vi "DisplayJson.vi"(11 "JSON String In":string="[{\"version\":\"1.0.0\",\"header\":{\"creationDate\":\"2022-06-03T00:00:00\",\"remarks\":\"\",\"serialNumber\":\"98172\",\"productNumber\":\"123021.1804\",\"productType\":\"PAA-9L\",\"pressureType\":2,\"productSeries\":\"9L\",\"compensatedTemperatureRange\":{\"min\":-10.0,\"max\":80.0,\"unit\":4},\"compensatedPressureRange\":{\"min\":0.0,\"max\":0.35,\"unit\":3},\"electricSupply\":{\"magnitude\":1.0,\"unit\":18},\"orderNumber\":9990266,\"orderPosition\":3,\"orderTargetDispatchDate\":\"2022-06-02T00:00:00+00:00\",\"customerName\":\"DemoData Inc.\",\"customerNumber\":12345678,\"customerOrderNumber\":\"Cust-9990266-123\",\"customerReferenceNumber\":\"\",\"customerProductT...") -> ()   [LabVIEW 2017] (continued)
magnitude\":59.8651,\"unit\":4},\"supply\":{\"magnitude\":1.0,\"unit\":18}},\"raw\":{\"signal\":{\"magnitude\":64.467783206,\"unit\":22},\"bridgeResistance\":{\"magnitude\":3852.3455546,\"unit\":28}},\"compensated\":{\"mathematicalModels\":{\"MM0123\":{\"pressure\":{\"output\":{\"magnitude\":0.349985,\"unit\":3},\"error\":{\"magnitude\":-0.0019717653,\"unit\":7}},\"temperature\":{\"output\":{\"magnitude\":59.9371,\"unit\":4},\"error\":{\"magnitude\":0.071974206,\"unit\":4}}}}}},{\"reference\":\"F_12300_XX_0000098765\",\"environmentTarget\":{\"pressure\":{\"magnitude\":0.03,\"unit\":3},\"temperature\":{\"magnitude\":80.0,\"unit\":4}},\"environment\":{\"pressure\":{\"magnitude\":0.0299952,\"unit\":3},\"temperature\":{\"magnitude\":79.9513,\"unit\":4},\"supply\":{\"magnitude\":1.0,\"unit\":18}},\"raw\":{\"signal\":{\"magnitude\":20.009624769,\"unit\":22},\"bridgeResistance\":{\"magnitude\":4076.9393183,\"unit\":28}},\"compensated\":{\"mathematicalModels\":{\"MM0123\":{\"pressure\":{\"output\":{\"magnitude\":0.0300118,\"unit\":3},\"error\":{\"magnitude\":0.0047428932,\"unit\":7}},\"temperature\":{\"output\":{\"magnitude\":80.0429,\"unit\":4},\"error\":{\"magnitude\":0.091598008,\"unit\":4}}}}}},{\"reference\":\"F_12300_XX_0000098765\",\"environmentTarget\":{\"pressure\":{\"magnitude\":0.11,\"unit\":3},\"temperature\":{\"magnitude\":80.0,\"unit\":4}},\"environment\":{\"pressure\":{\"magnitude\":0.110003,\"unit\":3},\"temperature\":{\"magnitude\":79.9513,\"unit\":4},\"supply\":{\"magnitude\":1.0,\"unit\":18}},\"raw\":{\"signal\":{\"magnitude\":31.586032437,\"unit\":22},\"bridgeResistance\":{\"magnitude\":4072.4664155,\"unit\":28}},\"compensated\":{\"mathematicalModels\":{\"MM0123\":{\"pressure\":{\"output\":{\"magnitude\":0.109961,\"unit\":3},\"error\":{\"magnitude\":-0.011912582,\"unit\":7}},\"temperature\":{\"output\":{\"magnitude\":80.0462,\"unit\":4},\"error\":{\"magnitude\":0.094860315,\"unit\":4}}}}}},{\"reference\":\"F_12300_XX_0000098765\",\"environmentTarget\":{\"pressure\":{\"magnitude\":0.19,\"unit\":3},\"temperature\":{\"magnitude\":80.0,\"unit\":4}},\"environment\":{\"pressure\":{\"magnitude\":0.189995,\"unit\":3},\"temperature\":{\"magnitude\":79.9513,\"unit\":4},\"supply\":{\"magnitude\":1.0,\"unit\":18}},\"raw\":{\"signal\":{\"magnitude\":43.149115129,\"unit\":22},\"bridgeResistance\":{\"magnitude\":4068.082853,\"unit\":28}},\"compensated\":{\"mathematicalModels\":{\"MM0123\":{\"pressure\":{\"output\":{\"magnitude\":0.190002,\"unit\":3},\"error\":{\"magnitude\":0.0020917834,\"unit\":7}},\"temperature\":{\"output\":{\"magnitude\":80.0546,\"unit\":4},\"error\":{\"magnitude\":0.10324897,\"unit\":4}}}}}},{\"reference\":\"F_12300_XX_0000098765\",\"environmentTarget\":{\"pressure\":{\"magnitude\":0.27,\"unit\":3},\"temperature\":{\"magnitude\":80.0,\"unit\":4}},\"environment\":{\"pressure\":{\"magnitude\":0.270005,\"unit\":3},\"temperature\":{\"magnitude\":79.9513,\"unit\":4},\"supply\":{\"magnitude\":1.0,\"unit\":18}},\"raw\":{\"signal\":{\"magnitude\":54.683724116,\"unit\":22},\"bridgeResistance\":{\"magnitude\":4063.7153683,\"unit\":28}},\"compensated\":{\"mathematicalModels\":{\"MM0123\":{\"pressure\":{\"output\":{\"magnitude\":0.270035,\"unit\":3},\"error\":{\"magnitude\":0.0086059364,\"unit\":7}},\"temperature\":{\"output\":{\"magnitude\":80.0606,\"unit\":4},\"error\":{\"magnitude\":0.10926909,\"unit\":4}}}}}},{\"reference\":\"F_12300_XX_0000098765\",\"environmentTarget\":{\"pressure\":{\"magnitude\":0.35,\"unit\":3},\"temperature\":{\"magnitude\":80.0,\"unit\":4}},\"environment\":{\"pressure\":{\"magnitude\":0.350001,\"unit\":3},\"temperature\":{\"magnitude\":79.9513,\"unit\":4},\"supply\":{\"magnitude\":1.0,\"unit\":18}},\"raw\":{\"signal\":{\"magnitude\":66.178985809,\"unit\":22},\"bridgeResistance\":{\"magnitude\":4059.3928573,\"unit\":28}},\"compensated\":{\"mathematicalModels\":{\"MM0123\":{\"pressure\":{\"output\":{\"magnitude\":0.349984,\"unit\":3},\"error\":{\"magnitude\":-0.0048720874,\"unit\":7}},\"temperature\":{\"output\":{\"magnitude\":80.0663,\"unit\":4},\"error\":{\"magnitude\":0.114986,\"unit\":4}}}}}}]},{\"version\":\"1.0.0\",\"header\":{\"creationDate\":\"2022-06-03T00:00:00\",\"remarks\":\"\",\"serialNumber\":\"98030\",\"productNumber\":\"123021.1804\",\"productType\":\"PAA-9L\",\"pressureType\":2,\"productSeries\":\"9L\",\"compensatedTemperatureRange\":{\"min\":-10.0,\"max\":80.0,\"unit\":4},\"compensatedPressureRange\":{\"min\":0.0,\"max\":0.35,\"unit\":3},\"electricSupply\":{\"magnitude\":1.0,\"unit\":18},\"orderNumber\":9990266,\"orderPosition\":3,\"orderTargetDispatchDate\":\"2022-06-02T00:00:00+00:00\",\"customerName\":\"DemoData Inc.\",\"customerNumber\":12345678,\"customerOrderNumber\":\"Cust-9990266-123\",\"customerReferenceNumber\":\"\",\"customerProductType\":\"123021-1804 Rev.AA\"},\"compensationMethods\":{\"mathematicalModels\":{\"MM0123\":{\"modelType\":\"MM0123\",\"productNumber\":\"000000.0000\",\"compensatedTemperatureRange\":{\"min\":-10.0,\"max\":80.0,\"unit\":4},\"compensatedPressureRange\":{\"min\":0.0,\"max\":0.35,\"unit\":3},\"electricSupply\":{\"magnitude\":1.0,\"unit\":18},\"parts\":{\"pressure\":{\"inputs\":[\"Sig\",\"R\"],\"output\":\"P\",\"description\":\"P = f(Sig,R)\",\"coefficients\":[[3.91051610792,-0.00396303697808,1.49281608913E-06,-2.51964333732E-10,1.59626202738E-14],[-0.118371633509,0.000126551102362,-4.7723277619E-08,7.99004276927E-12,-5.02310435685E-16],[-0.000301862256289,3.5208950299E-07,-1.51215801138E-10,2.85596859923E-14,-2.00879963271E-18]]},\"temperature\":{\"inputs\":[\"R\",\"Sig\"],\"output\":\"T\",\"description\":\"T = f(R,Sig)\",\"coefficients\":[[-7800.26845732,-7.96154289458,0.0704333830142],[7.62753908696,0.00996321268213,-8.05974057259E-05],[-0.00286192784163,-4.51133002231E-06,3.42637785226E-08],[4.86703234067E-07,8.89561295675E-10,-6.42476105441E-12],[-3.12400283304E-11,-6.46081048648E-14,4.48929986852E-16]]}}}}},\"measurements\":[{\"reference\":\"F_12300_XX_0000098765\",\"environmentTarget\":{\"pressure\":{\"magnitude\":0.03,\"unit\":3},\"temperature\":{\"magnitude\":-10.0,\"unit\":4}},\"environment\":{\"pressure\":{\"magnitude\":0.0300053,\"unit\":3},\"temperature\":{\"magnitude\":-10.7286,\"unit\":4},\"supply\":{\"magnitude\":1.0,\"unit\":18}},\"raw\":{\"signal\":{\"magnitude\":14.318461418,\"unit\":22},\"bridgeResistance\":{\"magnitude\":3289.5907634,\"unit\":28}},\"compensated\":{\"mathematicalModels\":{\"MM0123\":{\"pressure\":{\"output\":{\"magnitude\":0.0300169,\"unit\":3},\"error\":{\"magnitude\":0.0033129561,\"unit\":7}},\"temperature\":{\"output\":{\"magnitude\":-10.8169,\"unit\":4},\"error\":{\"magnitude\":-0.089267989,\"unit\":4}}}}}},{\"reference\":\"F_12300_XX_0000098765\",\"environmentTarget\":{\"pressure\":{\"magnitude\":0.11,\"unit\":3},\"temperature\":{\"magnitude\":-10.0,\"unit\":4}},\"environment\":{\"pressure\":{\"magnitude\":0.10999,\"unit\":3},\"temperature\":{\"magnitude\":-10.7286,\"unit\":4},\"supply\":{\"magnitude\":1.0,\"unit\":18}},\"raw\":{\"signal\":{\"magnitude\":25.459617511,\"unit\":22},\"bridgeResistance\":{\"magnitude\":3284.2812107,\"unit\":28}},\"compensated\":{\"mathematicalModels\":{\"MM0123\":{\"pressure\":{\"output\":{\"magnitude\":0.109962,\"unit\":3},\"error\":{\"magnitude\":-0.0079150781,\"unit\":7}},\"temperature\":{\"output\":{\"magnitude\":-10.8249,\"unit\":4},\"error\":{\"magnitude\":-0.096259313,\"unit\":4}}}}}},{\"reference\":\"F_12300_XX_0000098765\",\"environmentTarget\":{\"pressure\":{\"magnitude\":0.19,\"unit\":3},\"temperature\":{\"magnitude\":-10.0,\"unit\":4}},\"environment\":{\"pressure\":{\"magnitude\":0.190001,\"unit\":3},\"temperature\":{\"magnitude\":-10.7286,\"unit\":4},\"supply\":{\"magnitude\":1.0,\"unit\":18}},\"raw\":{\"signal\":{\"magnitude\":36.571102004,\"unit\":22},\"bridgeResistance\":{\"magnitude\":3280.172315,\"unit\":28}},\"compensated\":{\"mathematicalModels\":{\"MM0123\":{\"pressure\":{\"output\":{\"magnitude\":0.190009,\"unit\":3},\"error\":{\"magnitude\":0.0024238375,\"unit\":7}},\"temperature\":{\"output\":{\"magnitude\":-10.8183,\"unit\":4},\"error\":{\"magnitude\":-0.089645595,\"unit\":4}}}}}},{\"reference\":\"F_12300_XX_0000098765\",\"environmentTarget\":{\"pressure\":{\"magnitude\":0.27,\"unit\":3},\"temperature\":{\"magnitude\":-10.0,\"unit\":4}},\"environment\":{\"pressure\":{\"magnitude\":0.270006,\"unit\":3},\"temperature\":{\"magnitude\":-10.7286,\"unit\":4},\"supply\":{\"magnitude\":1.0,\"unit\":18}},\"raw\":{\"signal\":{\"magnitude\":47.63478106,\"unit\":22},\"bridgeResistance\":{\"magnitude\":3276.1315246,\"unit\":28}},\"compensated\":{\"mathematicalModels\":{\"MM0123\":{\"pressure\":{\"output\":{\"magnitude\":0.270034,\"unit\":3},\"error\":{\"magnitude\":0.0080862094,\"unit\":7}},\"temperature\":{\"output\":{\"magnitude\":-10.8182,\"unit\":4},\"error\":{\"magnitude\":-0.089598768,\"unit\":4}}}}}},{\"reference\":\"F_12300_XX_0000098765\",\"environmentTarget\":{\"pressure\":{\"magnitude\":0.35,\"unit\":3},\"temperature\":{\"magnitude\":-10.0,\"unit\":4}},\"environment\":{\"pressure\":{\"magnitude\":0.35,\"unit\":3},\"temperature\":{\"magnitude\":-10.7286,\"unit\":4},\"supply\":{\"magnitude\":1.0,\"unit\":18}},\"raw\":{\"signal\":{\"magnitude\":58.644972732,\"unit\":22},\"bridgeResistance\":{\"magnitude\":3272.1742491,\"unit\":28}},\"compensated\":{\"mathematicalModels\":{\"MM0123\":{\"pressure\":{\"output\":{\"magnitude\":0.349995,\"unit\":3},\"error\":{\"magnitude\":-0.0015198512,\"unit\":7}},\"temperature\":{\"output\":{\"magnitude\":-10.823,\"unit\":4},\"error\":{\"magnitude\":-0.094366794,\"unit\":4}}}}}},{\"reference\":\"F_12300_XX_0000098765\",\"environmentTarget\":{\"pressure\":{\"magnitude\":0.03,\"unit\":3},\"temperature\":{\"magnitude\":0.0,\"unit\":4}},\"environment\":{\"pressure\":{\"magnitude\":0.0299991,\"unit\":3},\"temperature\":{\"magnitude\":-0.629962,\"unit\":4},\"supply\":{\"magnitude\":1.0,\"unit\":18}},\"raw\":{\"signal\":{\"magnitude\":14.719120521,\"unit\":22},\"bridgeResistance\":{\"magnitude\":3358.468982,\"unit\":28}},\"compensated\":{\"mathematicalModels\":{\"MM0123\":{\"pressure\":{\"output\":{\"magnitude\":0.0300133,\"unit\":3},\"error\":{\"magnitude\":0.0040708695,\"unit\":7}},\"temperature\":{\"output\":{\"magnitude\":-0.731686,\"unit\":4},\"error\":{\"magnitude\":-0.10172384,\"unit\":4}}}}}},{\"reference\":\"F_12300_XX_0000098765\",\"environmentTarget\":{\"pressure\":{\"magnitude\":0.11,\"unit\":3},\"temperature\":{\"magnitude\":0.0,\"unit\":4}},\"environment\":{\"pressure\":{\"magnitude\":0.110012,\"unit\":3},\"temperature\":{\"magnitude\":-0.629962,\"unit\":4},\"supply\":{\"magnitude\":1.0,\"unit\":18}},\"raw\":{\"signal\":{\"magnitude\":25.832280563,\"unit\":22},\"bridgeResistance\":{\"magnitude\":3354.2253146,\"unit\":28}},\"compensated\":{\"mathematicalModels\":{\"MM0123\":{\"pressure\":{\"output\":{\"magnitude\":0.109979,\"unit\":3},\"error\":{\"magnitude\":-0.0093436435,\"unit\":7}},\"temperature\":{\"output\":{\"magnitude\":-0.731795,\"unit\":4},\"error\":{\"magnitude\":-0.10183319,\"unit\":4}}}}}},{\"reference\":\"F_12300_XX_0000098765\",\"environmentTarget\":{\"pressure\":{\"magnitude\":0.19,\"unit\":3},\"temperature\":{\"magnitude\":0.0,\"unit\":4}},\"environment\":{\"pressure\":{\"magnitude\":0.190005,\"unit\":3},\"temperature\":{\"magnitude\":-0.629962,\"unit\":4},\"supply\":{\"magnitude\":1.0,\"unit\":18}},\"raw\":{\"signal\":{\"magnitude\":36.911420503,\"unit\":22},\"bridgeResistance\":{\"magnitude\":3350.0635874,\"unit\":28}},\"compensated\":{\"mathematicalModels\":{\"MM0123\":{\"pressure\":{\"output\":{\"magnitude\":0.190007,\"unit\":3},\"error\":{\"magnitude\":0.00070119695,\"unit\":7}},\"temperature\":{\"output\":{\"magnitude\":-0.733503,\"unit\":4},\"error\":{\"magnitude\":-0.10354162,\"unit\":4}}}}}},{\"reference\":\"F_12300_XX_0000098765\",\"environmentTarget\":{\"pressure\":{\"magnitude\":0.27,\"unit\":3},\"temperature\":{\"magnitude\":0.0,\"unit\":4}},\"environment\":{\"pressure\":{\"magnitude\":0.270005,\"unit\":3},\"temperature\":{\"magnitude\":-0.629962,\"unit\":4},\"supply\":{\"magnitude\":1.0,\"unit\":18}},\"raw\":{\"signal\":{\"magnitude\":47.944742767,\"unit\":22},\"bridgeResistance\":{\"magnitude\":3345.9709897,\"unit\":28}},\"compensated\":{\"mathematicalModels\":{\"MM0123\":{\"pressure\":{\"output\":{\"magnitude\":0.270014,\"unit\":3},\"error\":{\"magnitude\":0.0025000508,\"unit\":7}},\"temperature\":{\"output\":{\"magnitude\":-0.739521,\"unit\":4},\"error\":{\"magnitude\":-0.10955897,\"unit\":4}}}}}},{\"reference\":\"F_12300_XX_0000098765\",\"environmentTarget\":{\"pressure\":{\"magnitude\":0.35,\"unit\":3},\"temperature\":{\"magnitude\":0.0,\"unit\":4}},\"environment\":{\"pressure\":{\"magnitude\":0.350001,\"unit\":3},\"temperature\":{\"magnitude\":-0.629962,\"unit\":4},\"supply\":{\"magnitude\":1.0,\"unit\":18}},\"raw\":{\"signal\":{\"magnitude\":58.929179764,\"unit\":22},\"bridgeResistance\":{\"magnitude\":3342.0076022,\"unit\":28}},\"compensated\":{\"mathematicalModels\":{\"MM0123\":{\"pressure\":{\"output\":{\"magnitude\":0.349974,\"unit\":3},\"error\":{\"magnitude\":-0.0077921223,\"unit\":7}},\"temperature\":{\"output\":{\"magnitude\":-0.741948,\"unit\":4},\"error\":{\"magnitude\":-0.1129859,\"unit\":4}}}}}},{\"reference\":\"F_12300_XX_0000098765\",\"environmentTarget\":{\"pressure\":{\"magnitude\":0.03,\"unit\":3},\"temperature\":{\"magnitude\":20.0,\"unit\":4}},\"environment\":{\"pressure\":{\"magnitude\":0.0300045,\"unit\":3},\"temperature\":{\"magnitude\":19.5509,\"unit\":4},\"supply\":{\"magnitude\":1.0,\"unit\":18}},\"raw\":{\"signal\":{\"magnitude\":15.541489722,\"unit\":22},\"bridgeResistance\":{\"magnitude\":3515.4448937,\"unit\":28}},\"compensated\":{\"mathematicalModels\":{\"MM0123\":{\"pressure\":{\"output\":{\"magnitude\":0.0300159,\"unit\":3},\"error\":{\"magnitude\":0.003267515,\"unit\":7}},\"temperature\":{\"output\":{\"magnitude\":19.5547,\"unit\":4},\"error\":{\"magnitude\":0.0038291876,\"unit\":4}}}}}},{\"reference\":\"F_12300_XX_0000098765\",\"environmentTarget\":{\"pressure\":{\"magnitude\":0.11,\"unit\":3},\"temperature\":{\"magnitude\":20.0,\"unit\":4}},\"environment\":{\"pressure\":{\"magnitude\":0.109996,\"unit\":3},\"temperature\":{\"magnitude\":19.5509,\"unit\":4},\"supply\":{\"magnitude\":1.0,\"unit\":18}},\"raw\":{\"signal\":{\"magnitude\":26.644230328,\"unit\":22},\"bridgeResistance\":{\"magnitude\":3511.171863,\"unit\":28}},\"compensated\":{\"mathematicalModels\":{\"MM0123\":{\"pressure\":{\"output\":{\"magnitude\":0.109975,\"unit\":3},\"error\":{\"magnitude\":-0.005894568,\"unit\":7}},\"temperature\":{\"output\":{\"magnitude\":19.5469,\"unit\":4},\"error\":{\"magnitude\":-0.0039398524,\"unit\":4}}}}}},{\"reference\":\"F_12300_XX_0000098765\",\"environmentTarget\":{\"pressure\":{\"magnitude\":0.19,\"unit\":3},\"temperature\":{\"magnitude\":20.0,\"unit\":4}},\"environment\":{\"pressure\":{\"magnitude\":0.189992,\"unit\":3},\"temperature\":{\"magnitude\":19.5509,\"unit\":4},\"supply\":{\"magnitude\":1.0,\"unit\":18}},\"raw\":{\"signal\":{\"magnitude\":37.718116681,\"unit\":22},\"bridgeResistance\":{\"magnitude\":3507.0336187,\"unit\":28}},\"compensated\":{\"mathematicalModels\":{\"MM0123\":{\"pressure\":{\"output\":{\"magnitude\":0.190001,\"unit\":3},\"error\":{\"magnitude\":0.0026963766,\"unit\":7}},\"temperature\":{\"output\":{\"magnitude\":19.5474,\"unit\":4},\"error\":{\"magnitude\":-0.0034972219,\"unit\":4}}}}}},{\"reference\":\"F_12300_XX_0000098765\",\"environmentTarget\":{\"pressure\":{\"magnitude\":0.27,\"unit\":3},\"temperature\":{\"magnitude\":20.0,\"unit\":4}},\"environment\":{\"pressure\":{\"magnitude\":0.269996,\"unit\":3},\"temperature\":{\"magnitude\":19.5509,\"unit\":4},\"supply\":{\"magnitude\":1.0,\"unit\":18}},\"raw\":{\"signal\":{\"magnitude\":48.753140854,\"unit\":22},\"bridgeResistance\":{\"magnitude\":3502.9189005,\"unit\":28}},\"compensated\":{\"mathematicalModels\":{\"MM0123\":{\"pressure\":{\"output\":{\"magnitude\":0.270027,\"unit\":3},\"error\":{\"magnitude\":0.0087365389,\"unit\":7}},\"temperature\":{\"output\":{\"magnitude\":19.5419,\"unit\":4},\"error\":{\"magnitude\":-0.0089498086,\"unit\":4}}}}}},{\"reference\":\"F_12300_XX_0000098765\",\"environmentTarget\":{\"pressure\":{\"magnitude\":0.35,\"unit\":3},\"temperature\":{\"magnitude\":20.0,\"unit\":4}},\"environment\":{\"pressure\":{\"magnitude\":0.350008,\"unit\":3},\"temperature\":{\"magnitude\":19.5509,\"unit\":4},\"supply\":{\"magnitude\":1.0,\"unit\":18}},\"raw\":{\"signal\":{\"magnitude\":59.744665253,\"unit\":22},\"bridgeResistance\":{\"magnitude\":3498.9179563,\"unit\":28}},\"compensated\":{\"mathematicalModels\":{\"MM0123\":{\"pressure\":{\"output\":{\"magnitude\":0.350014,\"unit\":3},\"error\":{\"magnitude\":0.0016130378,\"unit\":7}},\"temperature\":{\"output\":{\"magnitude\":19.5411,\"unit\":4},\"error\":{\"magnitude\":-0.0098247912,\"unit\":4}}}}}},{\"reference\":\"F_12300_XX_0000098765\",\"environmentTarget\":{\"pressure\":{\"magnitude\":0.03,\"unit\":3},\"temperature\":{\"magnitude\":40.0,\"unit\":4}},\"environment\":{\"pressure\":{\"magnitude\":0.0300059,\"unit\":3},\"temperature\":{\"magnitude\":39.7284,\"unit\":4},\"supply\":{\"magnitude\":1.0,\"unit\":18}},\"raw\":{\"signal\":{\"magnitude\":16.399203422,\"unit\":22},\"bridgeResistance\":{\"magnitude\":3691.7829758,\"unit\":28}},\"compensated\":{\"mathematicalModels\":{\"MM0123\":{\"pressure\":{\"output\":{\"magnitude\":0.03002,\"unit\":3},\"error\":{\"magnitude\":0.0040225986,\"unit\":7}},\"temperature\":{\"output\":{\"magnitude\":39.7191,\"unit\":4},\"error\":{\"magnitude\":-0.009332642,\"unit\":4}}}}}},{\"reference\":\"F_12300_XX_0000098765\",\"environmentTarget\":{\"pressure\":{\"magnitude\":0.11,\"unit\":3},\"temperature\":{\"magnitude\":40.0,\"unit\":4}},\"environment\":{\"pressure\":{\"magnitude\":0.110005,\"unit\":3},\"temperature\":{\"magnitude\":39.7284,\"unit\":4},\"supply\":{\"magnitude\":1.0,\"unit\":18}},\"raw\":{\"signal\":{\"magnitude\":27.551585744,\"unit\":22},\"bridgeResistance\":{\"magnitude\":3687.567005,\"unit\":28}},\"compensated\":{\"mathematicalModels\":{\"MM0123\":{\"pressure\":{\"output\":{\"magnitude\":0.109972,\"unit\":3},\"error\":{\"magnitude\":-0.0093547176,\"unit\":7}},\"temperature\":{\"output\":{\"magnitude\":39.7199,\"unit\":4},\"error\":{\"magnitude\":-0.0085193451,\"unit\":4}}}}}},{\"reference\":\"F_12300_XX_0000098765\",\"environmentTarget\":{\"pressure\":{\"magnitude\":0.19,\"unit\":3},\"temperature\":{\"magnitude\":40.0,\"unit\":4}},\"environment\":{\"pressure\":{\"magnitude\":0.190006,\"unit\":3},\"temperature\":{\"magnitude\":39.7284,\"unit\":4},\"supply\":{\"magnitude\":1.0,\"unit\":18}},\"raw\":{\"signal\":{\"magnitude\":38.680898496,\"unit\":22},\"bridgeResistance\":{\"magnitude\":3683.382268,\"unit\":28}},\"compensated\":{\"mathematicalModels\":{\"MM0123\":{\"pressure\":{\"output\":{\"magnitude\":0.190004,\"unit\":3},\"error\":{\"magnitude\":-0.00055208464,\"unit\":7}},\"temperature\":{\"output\":{\"magnitude\":39.7185,\"unit\":4},\"error\":{\"magnitude\":-0.0099393531,\"unit\":4}}}}}},{\"reference\":\"F_12300_XX_0000098765\",\"environmentTarget\":{\"pressure\":{\"magnitude\":0.27,\"unit\":3},\"temperature\":{\"magnitude\":40.0,\"unit\":4}},\"environment\":{\"pressure\":{\"magnitude\":0.269995,\"unit\":3},\"temperature\":{\"magnitude\":39.7284,\"unit\":4},\"supply\":{\"magnitude\":1.0,\"unit\":18}},\"raw\":{\"signal\":{\"magnitude\":49.772956046,\"unit\":22},\"bridgeResistance\":{\"magnitude\":3679.236034,\"unit\":28}},\"compensated\":{\"mathematicalModels\":{\"MM0123\":{\"pressure\":{\"output\":{\"magnitude\":0.270014,\"unit\":3},\"error\":{\"magnitude\":0.0054525253,\"unit\":7}},\"temperature\":{\"output\":{\"magnitude\":39.715,\"unit\":4},\"error\":{\"magnitude\":-0.013413052,\"unit\":4}}}}}},{\"reference\":\"F_12300_XX_0000098765\",\"environmentTarget\":{\"pressure\":{\"magnitude\":0.35,\"unit\":3},\"temperature\":{\"magnitude\":40.0,\"unit\":4}},\"environment\":{\"pressure\":{\"magnitude\":0.349999,\"unit\":3},\"temperature\":{\"magnitude\":39.7284,\"unit\":4},\"supply\":{\"magnitude\":1.0,\"unit\":18}},\"raw\":{\"signal\":{\"magnitude\":60.824279525,\"unit\":22},\"bridgeResistance\":{\"magnitude\":3675.1754657,\"unit\":28}},\"compensated\":{\"mathematicalModels\":{\"MM0123\":{\"pressure\":{\"output\":{\"magnitude\":0.349975,\"unit\":3},\"error\":{\"magnitude\":-0.0069275504,\"unit\":7}},\"temperature\":{\"output\":{\"magnitude\":39.7144,\"unit\":4},\"error\":{\"magnitude\":-0.013980514,\"unit\":4}}}}}},{\"reference\":\"F_12300_XX_0000098765\",\"environmentTarget\":{\"pressure\":{\"magnitude\":0.03,\"unit\":3},\"temperature\":{\"magnitude\":60.0,\"unit\":4}},\"environment\":{\"pressure\":{\"magnitude\":0.029997,\"unit\":3},\"temperature\":{\"magnitude\":59.8651,\"unit\":4},\"supply\":{\"magnitude\":1.0,\"unit\":18}},\"raw\":{\"signal\":{\"magnitude\":17.318985526,\"unit\":22},\"bridgeResistance\":{\"magnitude\":3894.8381412,\"unit\":28}},\"compensated\":{\"mathematicalModels\":{\"MM0123\":{\"pressure\":{\"output\":{\"magnitude\":0.0300115,\"unit\":3},\"error\":{\"magnitude\":0.0041449051,\"unit\":7}},\"temperature\":{\"output\":{\"magnitude\":59.9209,\"unit\":4},\"error\":{\"magnitude\":0.055772163,\"unit\":4}}}}}},{\"reference\":\"F_12300_XX_0000098765\",\"environmentTarget\":{\"pressure\":{\"magnitude\":0.11,\"unit\":3},\"temperature\":{\"magnitude\":60.0,\"unit\":4}},\"environment\":{\"pressure\":{\"magnitude\":0.110005,\"unit\":3},\"temperature\":{\"magnitude\":59.8651,\"unit\":4},\"supply\":{\"magnitude\":1.0,\"unit\":18}},\"raw\":{\"signal\":{\"magnitude\":28.560738175,\"unit\":22},\"bridgeResistance\":{\"magnitude\":3890.5168751,\"unit\":28}},\"compensated\":{\"mathematicalModels\":{\"MM0123\":{\"pressure\":{\"output\":{\"magnitude\":0.109976,\"unit\":3},\"error\":{\"magnitude\":-0.0083491294,\"unit\":7}},\"temperature\":{\"output\":{\"magnitude\":59.9215,\"unit\":4},\"error\":{\"magnitude\":0.056345671,\"unit\":4}}}}}},{\"reference\":\"F_12300_XX_0000098765\",\"environmentTarget\":{\"pressure\":{\"magnitude\":0.19,\"unit\":3},\"temperature\":{\"magnitude\":60.0,\"unit\":4}},\"environment\":{\"pressure\":{\"magnitude\":0.189999,\"unit\":3},\"temperature\":{\"magnitude\":59.8651,\"unit\":4},\"supply\":{\"magnitude\":1.0,\"unit\":18}},\"raw\":{\"signal\":{\"magnitude\":39.782303618,\"unit\":22},\"bridgeResistance\":{\"magnitude\":3876.2845989,\"unit\":28}},\"compensated\":{\"mathematicalModels\":{\"MM0123\":{\"pressure\":{\"output\":{\"magnitude\":0.190006,\"unit\":3},\"error\":{\"magnitude\":0.0020397825,\"unit\":7}},\"temperature\":{\"output\":{\"magnitude\":59.9253,\"unit\":4},\"error\":{\"magnitude\":0.060208763,\"unit\":4}}}}}},{\"reference\":\"F_12300_XX_0000098765\",\"environmentTarget\":{\"pressure\":{\"magnitude\":0.27,\"unit\":3},\"temperature\":{\"magnitude\":60.0,\"unit\":4}},\"environment\":{\"pressure\":{\"magnitude\":0.270006,\"unit\":3},\"temperature\":{\"magnitude\":59.8651,\"unit\":4},\"supply\":{\"magnitude\":1.0,\"unit\":18}},\"raw\":{\"signal\":{\"magnitude\":50.973169405,\"unit\":22},\"bridgeResistance\":{\"magnitude\":3872.0681903,\"unit\":28}},\"compensated\":{\"mathematicalModels\":{\"MM0123\":{\"pressure\":{\"output\":{\"magnitude\":0.270032,\"unit\":3},\"error\":{\"magnitude\":0.0074286071,\"unit\":7}},\"temperature\":{\"output\":{\"magnitude\":59.9248,\"unit\":4},\"error\":{\"magnitude\":0.059655478,\"unit\":4}}}}}},{\"reference\":\"F_12300_XX_0000098765\",\"environmentTarget\":{\"pressure\":{\"magnitude\":0.35,\"unit\":3},\"temperature\":{\"magnitude\":60.0,\"unit\":4}},\"environment\":{\"pressure\":{\"magnitude\":0.349998,\"unit\":3},\"temperature\":{\"magnitude\":59.8651,\"unit\":4},\"supply\":{\"magnitude\":1.0,\"unit\":18}},\"raw\":{\"signal\":{\"magnitude\":62.124890508,\"unit\":22},\"bridgeResistance\":{\"magnitude\":3867.9625543,\"unit\":28}},\"compensated\":{\"mathematicalModels\":{\"MM0123\":{\"pressure\":{\"output\":{\"magnitude\":0.349989,\"unit\":3},\"error\":{\"magnitude\":-0.0026296876,\"unit\":7}},\"temperature\":{\"output\":{\"magnitude\":59.9291,\"unit\":4},\"error\":{\"magnitude\":0.063999775,\"unit\":4}}}}}},{\"reference\":\"F_12300_XX_0000098765\",\"environmentTarget\":{\"pressure\":{\"magnitude\":0.03,\"unit\":3},\"temperature\":{\"magnitude\":80.0,\"unit\":4}},\"environment\":{\"pressure\":{\"magnitude\":0.0299903,\"unit\":3},\"temperature\":{\"magnitude\":79.9513,\"unit\":4},\"supply\":{\"magnitude\":1.0,\"unit\":18}},\"raw\":{\"signal\":{\"magnitude\":18.324177315,\"unit\":22},\"bridgeResistance\":{\"magnitude\":4092.9171617,\"unit\":28}},\"compensated\":{\"mathematicalModels\":{\"MM0123\":{\"pressure\":{\"output\":{\"magnitude\":0.0300078,\"unit\":3},\"error\":{\"magnitude\":0.0049996871,\"unit\":7}},\"temperature\":{\"output\":{\"magnitude\":80.0301,\"unit\":4},\"error\":{\"magnitude\":0.078723462,\"unit\":4}}}}}},{\"reference\":\"F_12300_XX_0000098765\",\"environmentTarget\":{\"pressure\":{\"magnitude\":0.11,\"unit\":3},\"temperature\":{\"magnitude\":80.0,\"unit\":4}},\"environment\":{\"pressure\":{\"magnitude\":0.110003,\"unit\":3},\"temperature\":{\"magnitude\":79.9513,\"unit\":4},\"supply\":{\"magnitude\":1.0,\"unit\":18}},\"raw\":{\"signal\":{\"magnitude\":29.678942571,\"unit\":22},\"bridgeResistance\":{\"magnitude\":4089.5493668,\"unit\":28}},\"compensated\":{\"mathematicalModels\":{\"MM0123\":{\"pressure\":{\"output\":{\"magnitude\":0.109963,\"unit\":3},\"error\":{\"magnitude\":-0.011497103,\"unit\":7}},\"temperature\":{\"output\":{\"magnitude\":80.0335,\"unit\":4},\"error\":{\"magnitude\":0.082171968,\"unit\":4}}}}}},{\"reference\":\"F_12300_XX_0000098765\",\"environmentTarget\":{\"pressure\":{\"magnitude\":0.19,\"unit\":3},\"temperature\":{\"magnitude\":80.0,\"unit\":4}},\"environment\":{\"pressure\":{\"magnitude\":0.190009,\"unit\":3},\"temperature\":{\"magnitude\":79.9513,\"unit\":4},\"supply\":{\"magnitude\":1.0,\"unit\":18}},\"raw\":{\"signal\":{\"magnitude\":41.023642697,\"unit\":22},\"bridgeResistance\":{\"magnitude\":4084.2532765,\"unit\":28}},\"compensated\":{\"mathematicalModels\":{\"MM0123\":{\"pressure\":{\"output\":{\"magnitude\":0.190014,\"unit\":3},\"error\":{\"magnitude\":0.0013437514,\"unit\":7}},\"temperature\":{\"output\":{\"magnitude\":80.0405,\"unit\":4},\"error\":{\"magnitude\":0.089169187,\"unit\":4}}}}}},{\"reference\":\"F_12300_XX_0000098765\",\"environmentTarget\":{\"pressure\":{\"magnitude\":0.27,\"unit\":3},\"temperature\":{\"magnitude\":80.0,\"unit\":4}},\"environment\":{\"pressure\":{\"magnitude\":0.270005,\"unit\":3},\"temperature\":{\"magnitude\":79.9513,\"unit\":4},\"supply\":{\"magnitude\":1.0,\"unit\":18}},\"raw\":{\"signal\":{\"magnitude\":52.340256366,\"unit\":22},\"bridgeResistance\":{\"magnitude\":4080.0085689,\"unit\":28}},\"compensated\":{\"mathematicalModels\":{\"MM0123\":{\"pressure\":{\"output\":{\"magnitude\":0.270037,\"unit\":3},\"error\":{\"magnitude\":0.0091649841,\"unit\":7}},\"temperature\":{\"output\":{\"magnitude\":80.0482,\"unit\":4},\"error\":{\"magnitude\":0.09689142,\"unit\":4}}}}}},{\"reference\":\"F_12300_XX_0000098765\",\"environmentTarget\":{\"pressure\":{\"magnitude\":0.35,\"unit\":3},\"temperature\":{\"magnitude\":80.0,\"unit\":4}},\"environment\":{\"pressure\":{\"magnitude\":0.350005,\"unit\":3},\"temperature\":{\"magnitude\":79.9513,\"unit\":4},\"supply\":{\"magnitude\":1.0,\"unit\":18}},\"raw\":{\"signal\":{\"magnitude\":63.622008536,\"unit\":22},\"bridgeResistance\":{\"magnitude\":4075.7753158,\"unit\":28}},\"compensated\":{\"mathematicalModels\":{\"MM0123\":{\"pressure\":{\"output\":{\"magnitude\":0.349989,\"unit\":3},\"error\":{\"magnitude\":-0.0045368461,\"unit\":7}},\"temperature\":{\"output\":{\"magnitude\":80.0525,\"unit\":4},\"error\":{\"magnitude\":0.1011257,\"unit\":4}}}}}}]},{\"version\":\"1.0.0\",\"header\":{\"creationDate\":\"2022-06-03T00:00:00\",\"remarks\":\"\",\"serialNumber\":\"98072\",\"productNumber\":\"123021.1804\",\"productType\":\"PAA-9L\",\"pressureType\":2,\"productSeries\":\"9L\",\"compensatedTemperatureRange\":{\"min\":-10.0,\"max\":80.0,\"unit\":4},\"compensatedPressureRange\":{\"min\":0.0,\"max\":0.35,\"unit\":3},\"electricSupply\":{\"magnitude\":1.0,\"unit\":18},\"orderNumber\":9990266,\"orderPosition\":3,\"orderTargetDispatchDate\":\"2022-06-02T00:00:00+00:00\",\"customerName\":\"DemoData Inc.\",\"customerNumber\":12345678,\"customerOrderNumber\":\"Cust-9990266-123\",\"customerReferenceNumber\":\"\",\"customerProductType\":\"123021-1804 Rev.AA\"},\"compensationMethods\":{\"mathematicalModels\":{\"MM0123\":{\"modelType\":\"MM0123\",\"productNumber\":\"000000.0000\",\"compensatedTemperatureRange\":{\"min\":-10.0,\"max\":80.0,\"unit\":4},\"compensatedPressureRange\":{\"min\":0.0,\"max\":0.35,\"unit\":3},\"electricSupply\":{\"magnitude\":1.0,\"unit\":18},\"parts\":{\"pressure\":{\"inputs\":[\"Sig\",\"R\"],\"output\":\"P\",\"description\":\"P = f(Sig,R)\",\"coefficients\":[[4.10922633276,-0.00414807894589,1.55291359634E-06,-2.60394730953E-10,1.63395585585E-14],[-0.11580899647,0.000123878160936,-4.66534054927E-08,7.7966608594E-12,-4.8908351259E-16],[-0.000277311308653,3.30087290084E-07,-1.44189007445E-10,2.76281444206E-14,-1.96749703066E-18]]},\"temperature\":{\"inputs\":[\"R\",\"Sig\"],\"output\":\"T\",\"description\":\"T = f(R,Sig)\",\"coefficients\":[[-8556.03173252,22.7683813432,-0.223589948568],[8.42233834981,-0.0236648601682,0.000242008132665],[-0.00317313001241,9.2564359989E-06,-9.81293998022E-08],[5.40636634824E-07,-1.61095011022E-09,1.76609248961E-11],[-3.47328620858E-11,1.05179671105E-13,-1.19018258963E-15]]}}}}},\"measurements\":[{\"reference\":\"F_12300_XX_0000098765\",\"environmentTarget\":{\"pressure\":{\"magnitude\":0.03,\"unit\":3},\"temperature\":{\"magnitude\":-10.0,\"unit\":4}},\"environment\":{\"pressure\":{\"magnitude\":0.0300053,\"unit\":3},\"temperature\":{\"magnitude\":-10.7286,\"unit\":4},\"supply\":{\"magnitude\":1.0,\"unit\":18}},\"raw\":{\"signal\":{\"magnitude\":16.373631558,\"unit\":22},\"bridgeResistance\":{\"magnitude\":3274.1307312,\"unit\":28}},\"compensated\":{\"mathematicalModels\":{\"MM0123\":{\"pressure\":{\"output\":{\"magnitude\":0.030016,\"unit\":3},\"error\":{\"magnitude\":0.0030697631,\"unit\":7}},\"temperature\":{\"output\":{\"magnitude\":-10.85,\"unit\":4},\"error\":{\"magnitude\":-0.12139579,\"unit\":4}}}}}},{\"reference\":\"F_12300_XX_0000098765\",\"environmentTarget\":{\"pressure\":{\"magnitude\":0.11,\"unit\":3},\"temperature\":{\"magnitude\":-10.0,\"unit\":4}},\"environment\":{\"pressure\":{\"magnitude\":0.110004,\"unit\":3},\"temperature\":{\"magnitude\":-10.7286,\"unit\":4},\"supply\":{\"magnitude\":1.0,\"unit\":18}},\"raw\":{\"signal\":{\"magnitude\":27.499085045,\"unit\":22},\"bridgeResistance\":{\"magnitude\":3269.9486611,\"unit\":28}},\"compensated\":{\"mathematicalModels\":{\"MM0123\":{\"pressure\":{\"output\":{\"magnitude\":0.109977,\"unit\":3},\"error\":{\"magnitude\":-0.0078346181,\"unit\":7}},\"temperature\":{\"output\":{\"magnitude\":-10.8516,\"unit\":4},\"error\":{\"magnitude\":-0.12299094,\"unit\":4}}}}}},{\"reference\":\"F_12300_XX_0000098765\",\"environmentTarget\":{\"pressure\":{\"magnitude\":0.19,\"unit\":3},\"temperature\":{\"magnitude\":-10.0,\"unit\":4}},\"environment\":{\"pressure\":{\"magnitude\":0.190008,\"unit\":3},\"temperature\":{\"magnitude\":-10.7286,\"unit\":4},\"supply\":{\"magnitude\":1.0,\"unit\":18}},\"raw\":{\"signal\":{\"magnitude\":38.594187568,\"unit\":22},\"bridgeResistance\":{\"magnitude\":3265.8615569,\"unit\":28}},\"compensated\":{\"mathematicalModels\":{\"MM0123\":{\"pressure\":{\"output\":{\"magnitude\":0.190016,\"unit\":3},\"error\":{\"magnitude\":0.0021559719,\"unit\":7}},\"temperature\":{\"output\":{\"magnitude\":-10.8527,\"unit\":4},\"error\":{\"magnitude\":-0.12408687,\"unit\":4}}}}}},{\"reference\":\"F_12300_XX_0000098765\",\"environmentTarget\":{\"pressure\":{\"magnitude\":0.27,\"unit\":3},\"temperature\":{\"magnitude\":-10.0,\"unit\":4}},\"environment\":{\"pressure\":{\"magnitude\":0.270002,\"unit\":3},\"temperature\":{\"magnitude\":-10.7286,\"unit\":4},\"supply\":{\"magnitude\":1.0,\"unit\":18}},\"raw\":{\"signal\":{\"magnitude\":49.644995408,\"unit\":22},\"bridgeResistance\":{\"magnitude\":3261.9033325,\"unit\":28}},\"compensated\":{\"mathematicalModels\":{\"MM0123\":{\"pressure\":{\"output\":{\"magnitude\":0.270033,\"unit\":3},\"error\":{\"magnitude\":0.0089344816,\"unit\":7}},\"temperature\":{\"output\":{\"magnitude\":-10.8497,\"unit\":4},\"error\":{\"magnitude\":-0.12104849,\"unit\":4}}}}}},{\"reference\":\"F_12300_XX_0000098765\",\"environmentTarget\":{\"pressure\":{\"magnitude\":0.35,\"unit\":3},\"temperature\":{\"magnitude\":-10.0,\"unit\":4}},\"environment\":{\"pressure\":{\"magnitude\":0.350001,\"unit\":3},\"temperature\":{\"magnitude\":-10.7286,\"unit\":4},\"supply\":{\"magnitude\":1.0,\"unit\":18}},\"raw\":{\"signal\":{\"magnitude\":60.646725805,\"unit\":22},\"bridgeResistance\":{\"magnitude\":3258.0099034,\"unit\":28}},\"compensated\":{\"mathematicalModels\":{\"MM0123\":{\"pressure\":{\"output\":{\"magnitude\":0.349998,\"unit\":3},\"error\":{\"magnitude\":-0.00096557513,\"unit\":7}},\"temperature\":{\"output\":{\"magnitude\":-10.8533,\"unit\":4},\"error\":{\"magnitude\":-0.12466322,\"unit\":4}}}}}},{\"reference\":\"F_12300_XX_0000098765\",\"environmentTarget\":{\"pressure\":{\"magnitude\":0.03,\"unit\":3},\"temperature\":{\"magnitude\":0.0,\"unit\":4}},\"environment\":{\"pressure\":{\"magnitude\":0.029996,\"unit\":3},\"temperature\":{\"magnitude\":-0.629962,\"unit\":4},\"supply\":{\"magnitude\":1.0,\"unit\":18}},\"raw\":{\"signal\":{\"magnitude\":16.862578495,\"unit\":22},\"bridgeResistance\":{\"magnitude\":3342.756408,\"unit\":28}},\"compensated\":{\"mathematicalModels\":{\"MM0123\":{\"pressure\":{\"output\":{\"magnitude\":0.0300137,\"unit\":3},\"error\":{\"magnitude\":0.0050461389,\"unit\":7}},\"temperature\":{\"output\":{\"magnitude\":-0.747116,\"unit\":4},\"error\":{\"magnitude\":-0.11715404,\"unit\":4}}}}}},{\"reference\":\"F_12300_XX_0000098765\",\"environmentTarget\":{\"pressure\":{\"magnitude\":0.11,\"unit\":3},\"temperature\":{\"magnitude\":0.0,\"unit\":4}},\"environment\":{\"pressure\":{\"magnitude\":0.110003,\"unit\":3},\"temperature\":{\"magnitude\":-0.629962,\"unit\":4},\"supply\":{\"magnitude\":1.0,\"unit\":18}},\"raw\":{\"signal\":{\"magnitude\":27.957038313,\"unit\":22},\"bridgeResistance\":{\"magnitude\":3338.6041995,\"unit\":28}},\"compensated\":{\"mathematicalModels\":{\"MM0123\":{\"pressure\":{\"output\":{\"magnitude\":0.109973,\"unit\":3},\"error\":{\"magnitude\":-0.008590796,\"unit\":7}},\"temperature\":{\"output\":{\"magnitude\":-0.751102,\"unit\":4},\"error\":{\"magnitude\":-0.12114035,\"unit\":4}}}}}},{\"reference\":\"F_12300_XX_0000098765\",\"environmentTarget\":{\"pressure\":{\"magnitude\":0.19,\"unit\":3},\"temperature\":{\"magnitude\":0.0,\"unit\":4}},\"environment\":{\"pressure\":{\"magnitude\":0.190003,\"unit\":3},\"temperature\":{\"magnitude\":-0.629962,\"unit\":4},\"supply\":{\"magnitude\":1.0,\"unit\":18}},\"raw\":{\"signal\":{\"magnitude\":39.021440482,\"unit\":22},\"bridgeResistance\":{\"magnitude\":3334.5716879,\"unit\":28}},\"compensated\":{\"mathematicalModels\":{\"MM0123\":{\"pressure\":{\"output\":{\"magnitude\":0.189997,\"unit\":3},\"error\":{\"magnitude\":-0.0017329314,\"unit\":7}},\"temperature\":{\"output\":{\"magnitude\":-0.748979,\"unit\":4},\"error\":{\"magnitude\":-0.11891684,\"unit\":4}}}}}},{\"reference\":\"F_12300_XX_0000098765\",\"environmentTarget\":{\"pressure\":{\"magnitude\":0.27,\"unit\":3},\"temperature\":{\"magnitude\":0.0,\"unit\":4}},\"environment\":{\"pressure\":{\"magnitude\":0.27,\"unit\":3},\"temperature\":{\"magnitude\":-0.629962,\"unit\":4},\"supply\":{\"magnitude\":1.0,\"unit\":18}},\"raw\":{\"signal\":{\"magnitude\":50.044626346,\"unit\":22},\"bridgeResistance\":{\"magnitude\":3330.5787605,\"unit\":28}},\"compensated\":{\"mathematicalModels\":{\"MM0123\":{\"pressure\":{\"output\":{\"magnitude\":0.27001,\"unit\":3},\"error\":{\"magnitude\":0.0029294245,\"unit\":7}},\"temperature\":{\"output\":{\"magnitude\":-0.752694,\"unit\":4},\"error\":{\"magnitude\":-0.1227319,\"unit\":4}}}}}},{\"reference\":\"F_12300_XX_0000098765\",\"environmentTarget\":{\"pressure\":{\"magnitude\":0.35,\"unit\":3},\"temperature\":{\"magnitude\":0.0,\"unit\":4}},\"environment\":{\"pressure\":{\"magnitude\":0.350003,\"unit\":3},\"temperature\":{\"magnitude\":-0.629962,\"unit\":4},\"supply\":{\"magnitude\":1.0,\"unit\":18}},\"raw\":{\"signal\":{\"magnitude\":61.021122571,\"unit\":22},\"bridgeResistance\":{\"magnitude\":3326.6776619,\"unit\":28}},\"compensated\":{\"mathematicalModels\":{\"MM0123\":{\"pressure\":{\"output\":{\"magnitude\":0.349971,\"unit\":3},\"error\":{\"magnitude\":-0.0090578229,\"unit\":7}},\"temperature\":{\"output\":{\"magnitude\":-0.755824,\"unit\":4},\"error\":{\"magnitude\":-0.1258618,\"unit\":4}}}}}},{\"reference\":\"F_12300_XX_0000098765\",\"environmentTarget\":{\"pressure\":{\"magnitude\":0.03,\"unit\":3},\"temperature\":{\"magnitude\":20.0,\"unit\":4}},\"environment\":{\"pressure\":{\"magnitude\":0.0300027,\"unit\":3},\"temperature\":{\"magnitude\":19.5509,\"unit\":4},\"supply\":{\"magnitude\":1.0,\"unit\":18}},\"raw\":{\"signal\":{\"magnitude\":17.891679398,\"unit\":22},\"bridgeResistance\":{\"magnitude\":3497.6078264,\"unit\":28}},\"compensated\":{\"mathematicalModels\":{\"MM0123\":{\"pressure\":{\"output\":{\"magnitude\":0.0300107,\"unit\":3},\"error\":{\"magnitude\":0.0022869073,\"unit\":7}},\"temperature\":{\"output\":{\"magnitude\":19.5396,\"unit\":4},\"error\":{\"magnitude\":-0.011302412,\"unit\":4}}}}}},{\"reference\":\"F_12300_XX_0000098765\",\"environmentTarget\":{\"pressure\":{\"magnitude\":0.11,\"unit\":3},\"temperature\":{\"magnitude\":20.0,\"unit\":4}},\"environment\":{\"pressure\":{\"magnitude\":0.109998,\"unit\":3},\"temperature\":{\"magnitude\":19.5509,\"unit\":4},\"supply\":{\"magnitude\":1.0,\"unit\":18}},\"raw\":{\"signal\":{\"magnitude\":28.97690627,\"unit\":22},\"bridgeResistance\":{\"magnitude\":3493.4343036,\"unit\":28}},\"compensated\":{\"mathematicalModels\":{\"MM0123\":{\"pressure\":{\"output\":{\"magnitude\":0.109975,\"unit\":3},\"error\":{\"magnitude\":-0.0065432526,\"unit\":7}},\"temperature\":{\"output\":{\"magnitude\":19.5328,\"unit\":4},\"error\":{\"magnitude\":-0.018029142,\"unit\":4}}}}}},{\"reference\":\"F_12300_XX_0000098765\",\"environmentTarget\":{\"pressure\":{\"magnitude\":0.19,\"unit\":3},\"temperature\":{\"magnitude\":20.0,\"unit\":4}},\"environment\":{\"pressure\":{\"magnitude\":0.189998,\"unit\":3},\"temperature\":{\"magnitude\":19.5509,\"unit\":4},\"supply\":{\"magnitude\":1.0,\"unit\":18}},\"raw\":{\"signal\":{\"magnitude\":40.037486344,\"unit\":22},\"bridgeResistance\":{\"magnitude\":3489.3845495,\"unit\":28}},\"compensated\":{\"mathematicalModels\":{\"MM0123\":{\"pressure\":{\"output\":{\"magnitude\":0.190011,\"unit\":3},\"error\":{\"magnitude\":0.0036599025,\"unit\":7}},\"temperature\":{\"output\":{\"magnitude\":19.5328,\"unit\":4},\"error\":{\"magnitude\":-0.018079197,\"unit\":4}}}}}},{\"reference\":\"F_12300_XX_0000098765\",\"environmentTarget\":{\"pressure\":{\"magnitude\":0.27,\"unit\":3},\"temperature\":{\"magnitude\":20.0,\"unit\":4}},\"environment\":{\"pressure\":{\"magnitude\":0.269994,\"unit\":3},\"temperature\":{\"magnitude\":19.5509,\"unit\":4},\"supply\":{\"magnitude\":1.0,\"unit\":18}},\"raw\":{\"signal\":{\"magnitude\":51.060372896,\"unit\":22},\"bridgeResistance\":{\"magnitude\":3485.3493548,\"unit\":28}},\"compensated\":{\"mathematicalModels\":{\"MM0123\":{\"pressure\":{\"output\":{\"magnitude\":0.27003,\"unit\":3},\"error\":{\"magnitude\":0.010231849,\"unit\":7}},\"temperature\":{\"output\":{\"magnitude\":19.5256,\"unit\":4},\"error\":{\"magnitude\":-0.025308152,\"unit\":4}}}}}},{\"reference\":\"F_12300_XX_0000098765\",\"environmentTarget\":{\"pressure\":{\"magnitude\":0.35,\"unit\":3},\"temperature\":{\"magnitude\":20.0,\"unit\":4}},\"environment\":{\"pressure\":{\"magnitude\":0.350011,\"unit\":3},\"temperature\":{\"magnitude\":19.5509,\"unit\":4},
